vi "MessageVSS_Simulator.vi"(9 "Array In":u8[](array[numeric]), 11 "Robot":T1 {"Vel Esquerda 3" format="%1_6f"; "Vel Esquerda 2" format="%1_6f"; "Vel Esquerda 1" format="%1_6f"; "Vel Direita 3" format="%1_6f"; "Vel Direita 2" format="%1_6f"; "Vel Direita 1" format="%1_6f"}) -> (1 "Array":u8[](array[numeric]))   [LabVIEW 2017]
uses:
  grSim/Viewer Robot Command.ctl
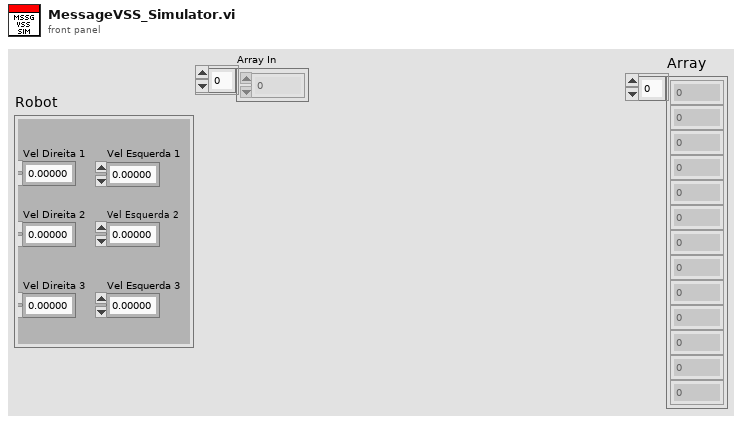
[diagram p1: front panel]
types:
  T1 = typedef "Viewer Robot Command.ctl" = cluster{"Vel Direita 1\n":dbl, "Vel Direita 2":dbl, "Vel Direita 3":dbl, "Vel Esquerda 1\n":dbl, "Vel Esquerda 2":dbl, "Vel Esquerda 3":dbl}
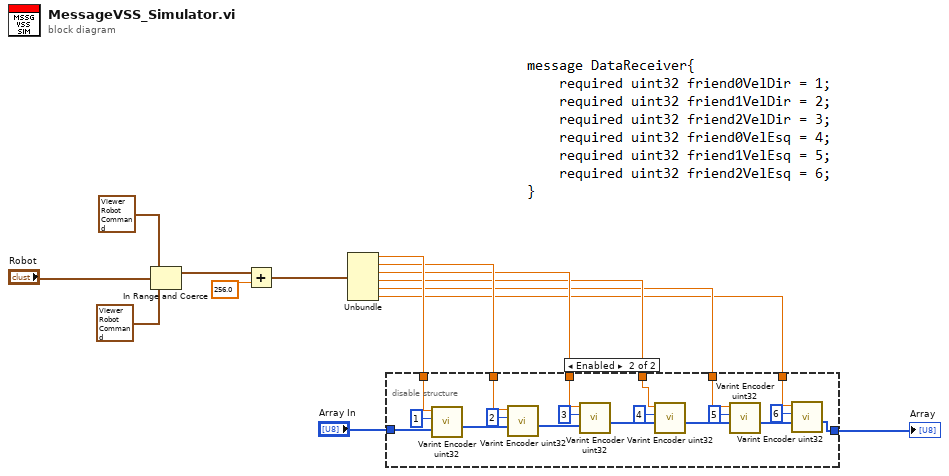
[diagram p0: block diagram]
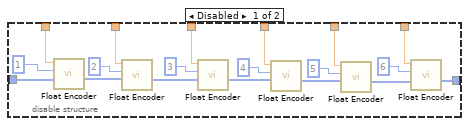
[diagram p2: hidden frame]
diagram:
  n1 = In Range and Coerce(upper limit=T1 {"Vel Direita 1\n"=255.0, "Vel Direita 2"=255.0, "Vel Direita 3"=255.0, "Vel Esquerda 1\n"=255.0, "Vel Esquerda 2"=255.0, "Vel Esquerda 3"=255.0}, x="Robot", lower limit=T1 {"Vel Direita 1\n"=-255.0, "Vel Direita 2"=-255.0, "Vel Direita 3"=-255.0, "Vel Esquerda 1\n"=-255.0, "Vel Esquerda 2"=-255.0, "Vel Esquerda 3"=-255.0}) -> (coerced(x)=w4:T1)  [unwired: 1 out]
  n2 = Add(x=w4, y=256.0) -> (x+y=w6:T1)
  n3 = Unbundle(w6) -> ("Vel Direita 1"=w13:dbl, "Vel Direita 2"=w11:dbl, "Vel Direita 3"=w10:dbl, "Vel Esquerda 1"=w9:dbl, "Vel Esquerda 2"=w8:dbl, "Vel Esquerda 3"=w7:dbl)
  n4 = disable-structure shown="Enabled" {
    disable-tunnel: "Array In" -> [w24 w52]
    disable-tunnel: w13 -> [w21 w40]
    disable-tunnel: [w20 w45] -> w12
    disable-tunnel: w11 -> [w19 w41]
    disable-tunnel: w10 -> [w18 w50]
    disable-tunnel: w9 -> [w17 w42]
    disable-tunnel: w8 -> [w16 w43]
    disable-tunnel: w7 -> [w15 w44]
    frame Disabled {
      n5 = call "Float Encoder.vi"("Array In"=w24, "Key"=u32 1, "Value"=w21) -> ("Array"=w23:u8[])  [unwired: 8 in]
      n6 = call "Float Encoder.vi"("Array In"=w23, "Key"=u32 2, "Value"=w19) -> ("Array"=w28:u8[])  [unwired: 8 in]
      n7 = call "Float Encoder.vi"("Array In"=w28, "Key"=u32 3, "Value"=w18) -> ("Array"=w27:u8[])  [unwired: 8 in]
      n8 = call "Float Encoder.vi"("Array In"=w27, "Key"=u32 4, "Value"=w17) -> ("Array"=w26:u8[])  [unwired: 8 in]
      n9 = call "Float Encoder.vi"("Array In"=w26, "Key"=u32 5, "Value"=w16) -> ("Array"=w25:u8[])  [unwired: 8 in]
      n10 = call "Float Encoder.vi"("Array In"=w25, "Key"=u32 6, "Value"=w15) -> ("Array"=w20:u8[])  [unwired: 8 in]
    }
    frame Enabled {
      n11 = call "Varint Encoder uint32.vi"("Array In"=w52, "Key"=u32 1, "Value"=w40) -> ("Array"=w51:u8[])  [unwired: 8 in]
      n12 = call "Varint Encoder uint32.vi"("Array In"=w51, "Key"=u32 2, "Value"=w41) -> ("Array"=w49:u8[])  [unwired: 8 in]
      n13 = call "Varint Encoder uint32.vi"("Array In"=w49, "Key"=u32 3, "Value"=w50) -> ("Array"=w48:u8[])  [unwired: 8 in]
      n14 = call "Varint Encoder uint32.vi"("Array In"=w48, "Key"=u32 4, "Value"=w42) -> ("Array"=w47:u8[])  [unwired: 8 in]
      n15 = call "Varint Encoder uint32.vi"("Array In"=w47, "Key"=u32 5, "Value"=w43) -> ("Array"=w46:u8[])  [unwired: 8 in]
      n16 = call "Varint Encoder uint32.vi"("Array In"=w46, "Key"=u32 6, "Value"=w44) -> ("Array"=w45:u8[])  [unwired: 8 in]
    }
  }
  "Array" <- w12
